vi "get module IDs from All Nodes Summary.vi"(8 "error in (no error)":errorcluster, 11 "summary":T1[](array[typedef])) -> (0 "error out":errorcluster, 3 "module IDs":string[](array[string]))   [LabVIEW 2013, in "Standard Editor.lvlib"]
uses:
  Standard Editor.lvlib
  <vilib>/NI/Configuration Framework/Node/Summary.ctl
  <vilib>/NI/Configuration Framework/Node/NISE_CEF_Node.lvclass
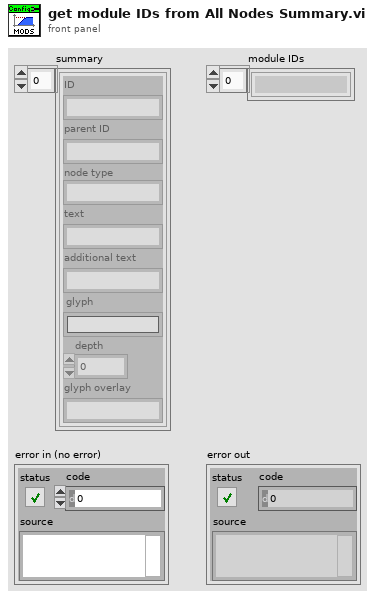
[diagram p1: front panel]
types:
  T1 = typedef "NISE_CEF_Node.lvclass/Summary.ctl" = cluster{"ID":string, "parent ID":string, "node type":string, "text":string, "additional text":string, "glyph":string, "depth":i32, "glyph overlay":string}
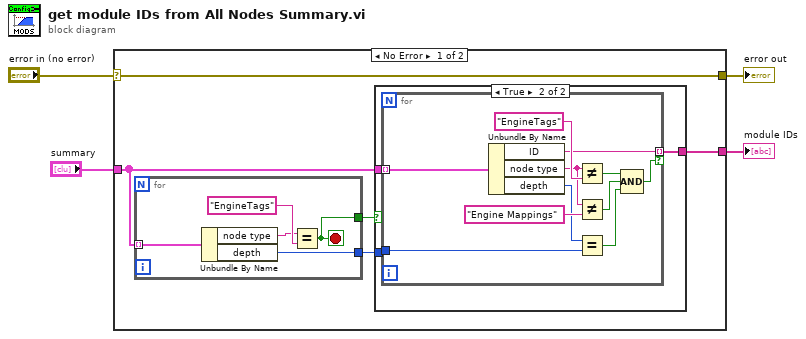
[diagram p0: block diagram]
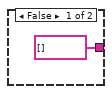
[diagram p2: hidden frame]
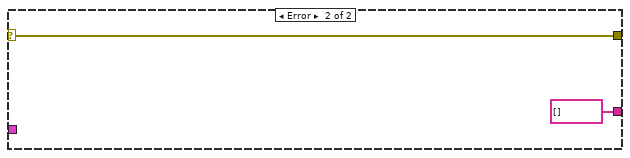
[diagram p3: hidden frame]
diagram:
  n1 = case shown="No Error" "error in (no error)" {
    selector: "error in (no error)" -> [w9 w31]
    tunnel: [w6 string[] []] -> w4
    tunnel: "summary" -> [w8 _]
    tunnel: [w9 w31] -> w1
    frame No Error {
      n2 = for {
        tunnel: w8 -> [w29] mode=indexing
        tunnel: [w26] -> w7
        tunnel: [w25] -> w5
        stop <- w25 stop-if-true
        n3 = Unbundle By Name(w29) -> ("node type"=w27:string, "depth"=w26:i32)
        n4 = Equal?(x=w27, y="EngineTags") -> (x = y?=w25:bool)
      }
      n5 = case shown="True" w5 {
        tunnel: w8 -> [_ w13]
        tunnel: w7 -> [_ w12]
        tunnel: [string[] [] w11] -> w6
        frame False {
        }
        frame True {
          n6 = for {
            tunnel: w13 -> [w24] mode=indexing
            tunnel: w12 -> [w19]
            tunnel: [w15] -> w11 mode=indexing if=w14
            n7 = Unbundle By Name(w24) -> ("ID"=w15:string, "node type"=w22:string, "depth"=w20:i32)
            n8 = Not Equal?(x=w22, y="EngineTags") -> (x != y?=w18:bool)
            n9 = Not Equal?(x=w22, y="Engine Mappings") -> (x != y?=w17:bool)
            n10 = Equal?(x=w20, y=w19) -> (x = y?=w16:bool)
            n11 = Compound Arithmetic op=AND(w18, w17, w16) -> (w14:bool)
          }
        }
      }
    }
    frame Error {
    }
  }
  "module IDs" <- w4
  "error out" <- w1
